vi "test_libssh2_sftp_init.vi"() -> ()   [LabVIEW 2017, in "integration_tests.lvlib"]
uses:
  integration_tests.lvlib
  support/support.lvlib
  libssh2/libssh2.lvlib
  <vilib>/PNR/Transparent Assertions/Transparent Assertions/Transparent Assertions.lvlib
panel:
  out "error out":errorcluster
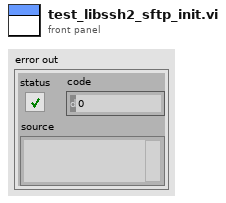
[diagram p1: front panel]
types:
  T1 = typedef "libssh2.lvlib/Session Refnum.ctl" = refnum<k1>
  T2 = typedef "libssh2.lvlib/SFTP Refnum.ctl" = refnum<k1>
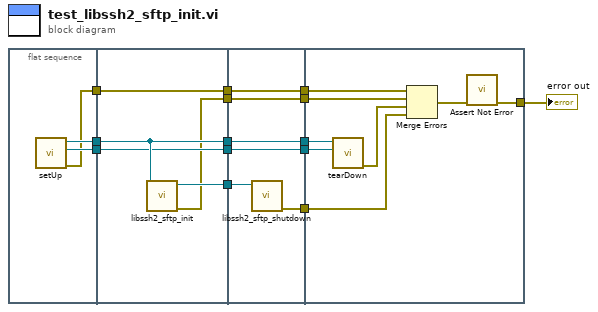
[diagram p0: block diagram]
diagram:
  n1 = flat-sequence {
    tunnel: [w17] -> w14
    tunnel: [w16] -> w13
    tunnel: [w15] -> w12
    tunnel: w14 -> [w22]
    tunnel: w13 -> [w21]
    tunnel: [w22] -> w10
    tunnel: [w21] -> w8
    tunnel: [w20] -> w6
    tunnel: [w19] -> w5
    tunnel: w12 -> [w19]
    tunnel: [w18] -> w2
    tunnel: w10 -> [w28]
    tunnel: [w28] -> w9
    tunnel: w8 -> [w27]
    tunnel: [w27] -> w7
    tunnel: w6 -> [w25]
    tunnel: w5 -> [w26]
    tunnel: [w26] -> w4
    tunnel: [w24] -> w3
    tunnel: w2 -> [w23]
    tunnel: [w23] -> w1
    tunnel: w9 -> [w36]
    tunnel: w7 -> [w35]
    tunnel: w4 -> [w34]
    tunnel: [w31] -> w11
    tunnel: w3 -> [w30]
    tunnel: w1 -> [w29]
    frame #0 {
      n2 = call "setUp.vi"() -> ("error out"=w15:errorcluster, "connection ID"=w16:refnum<k5>, "session"=w17:T1)  [unwired: 9 in]
    }
    frame #1 {
      n3 = call "libssh2_sftp_init.vi"("session"=w22) -> ("error out"=w18:errorcluster, "sftp"=w20:T2)  [unwired: 9 in]
    }
    frame #2 {
      n4 = call "libssh2_sftp_shutdown.vi"("sftp"=w25) -> ("error out"=w24:errorcluster)  [unwired: 10 in]
    }
    frame #3 {
      n5 = call "tearDown.vi"("connection ID"=w35, "session"=w36) -> ("error out"=w33:errorcluster)  [unwired: 9 in]
      n6 = Merge Errors(w34, w29, w33, w30) -> (w32:errorcluster)
      n7 = call <vilib>:"Assert Not Error.vi"("error in (no error)"=w32) -> ("error out"=w31:errorcluster)  [unwired: 10 in]
    }
  }
  "error out" <- w11
